vi "Populate Result.vi"(8 "error in (no error)":errorcluster, 11 "Numeric Limit Compare in":refnum<class "Numeric Limit Compare.lvclass">) -> (0 "error out":errorcluster, 3 "Numeric Limit Compare out":refnum<class "Numeric Limit Compare.lvclass">)   [LabVIEW 2018, in "Numeric Limit Compare.lvclass"]
doc: "This VI Gathers the information from the step and builds a result with it."
uses:
  Numeric Limit Compare.lvclass
  C:/Git/Danecca_Battery/sequencer/Prototype/classes/Step/Execution/Step.lvclass
  classes/Result/Result.lvclass
  classes/Step/Execution/Step Status.ctl
  Numeric Limit Compare.lvclass/Numeric Limit Compare.ctl
  classes/Step/Execution/Step.lvclass
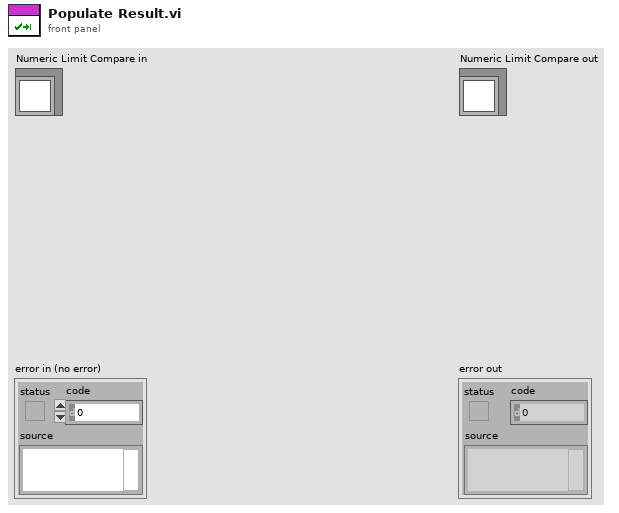
[diagram p1: front panel]
types:
  T1 = typedef "Step.lvclass/Step Status.ctl" = enum16{"Start", "Passed", "Failed", "Error", "Done", "Terminated", "Skipped", "Running"}
  T2 = typedef "Comparison Types.ctl" = enum16{"GELE (>=<=)", "GTLE(><=)", "GTLT(><)", "GELT(>=<)", "EQ(==)", "NE (!=)", "GT(>)", "LT(<)", "GE(>=)", "LE(<=)"}
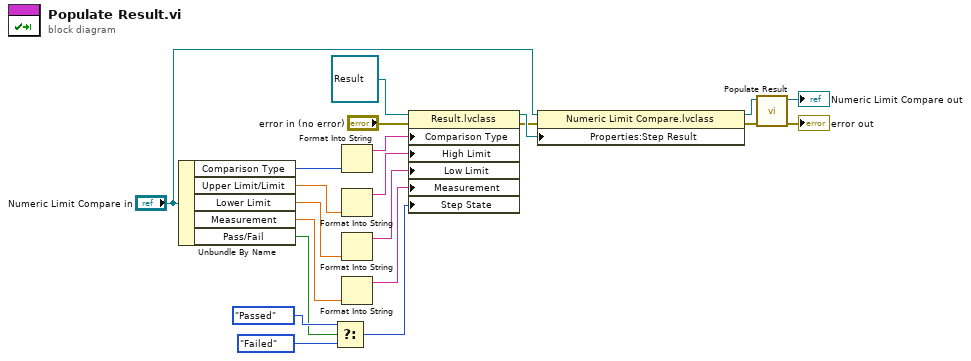
[diagram p0: block diagram]
diagram:
  n1 = Unbundle By Name("Numeric Limit Compare in") -> ("Comparison Type"=w16:T2, "Upper Limit/Limit"=w15:dbl, "Lower Limit"=w14:dbl, "Measurement"=w6:dbl, "Pass/Fail"=w2:bool)
  n2 = Select(t=Step_Status."Passed" ("Step State"), s=w2, f=Step_Status."Failed" ("Step State")) -> (s? t:f=w1:T1)
  n3 = Format Into String(w16) -> (resulting string=w13:string)  [unwired: 3 in, 1 out]
  n4 = Format Into String(w15) -> (resulting string=w12:string)  [unwired: 3 in, 1 out]
  n5 = Format Into String(w14) -> (resulting string=w11:string)  [unwired: 3 in, 1 out]
  n6 = Format Into String(w6) -> (resulting string=w5:string)  [unwired: 3 in, 1 out]
  n7 = property class="Result.lvclass"(reference=refnum<class "Result.lvclass"> refnum ("Result.lvclass"), error in="error in (no error)", "Comparison Type"=w13, "High Limit"=w12, "Low Limit"=w11, "Measurement"=w5, "Step State"=w1) -> (reference out=w19:refnum<class "Result.lvclass">, error out=w18:errorcluster)
  n8 = property class="Numeric Limit Compare.lvclass"(reference="Numeric Limit Compare in", error in=w18, "Properties:Step Result"=w19) -> (reference out=w10:refnum<class "Numeric Limit Compare.lvclass">, error out=w9:errorcluster)
  n9 = call-parent "Populate Result.vi"("error in (no error)"=w9, "Step in"=w10) -> ("error out"=→"error out":errorcluster, "Step out"=→"Numeric Limit Compare out":refnum<class "Numeric Limit Compare.lvclass">)  [unwired: 8 in]
